vi "SECoP-Initialize.vi"(8 "error in (no error)":errorcluster, 9 "Context ID (in)":string, 10 "show status window (GUI)":bool=TRUE, 11 "DLL path (in)":path) -> (0 "error out":errorcluster, 3 "DLL path (out)":T1)   [LabVIEW 2023, in "SECoP.lvlib"]
doc: "Call <b>\"SECoP-Initialize.vi\"</b> before use of any SHALL SEC-Node related functions. This loads and initialises external SHALL libraries.\n\n<b>DLL path (in)</b> input path to directory of SHALL libraries\n<b>DLL path (out)</b>) output of cluster to be used for other VIs\n<b>show status window (GUI)</b> boolean value to <b>show</b> (true) or <b>hide</b> (false) the status window on top right corner of display"
uses:
  SECoP.lvlib
  SECoP-libraries.ctl
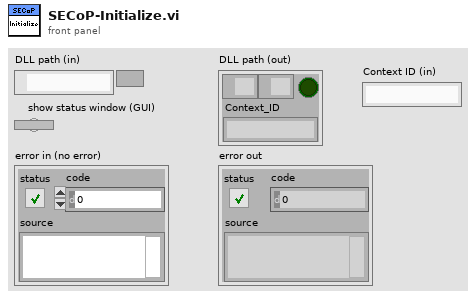
[diagram p1: front panel]
types:
  T1 = typedef "SECoP.lvlib/SECoP-libraries.ctl" = cluster{"serverDLL":path, "variantDLL":path, "cleanup_mode":bool, "Context_ID":string}
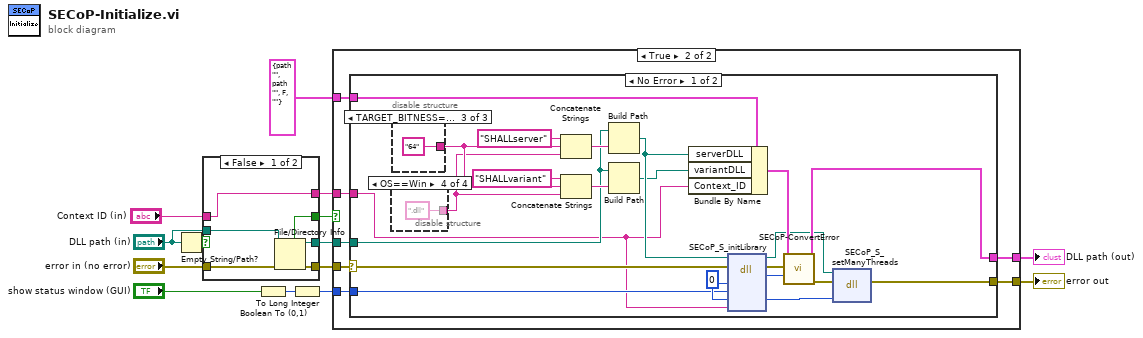
[diagram p0: block diagram]
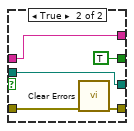
[diagram p2: hidden frame]
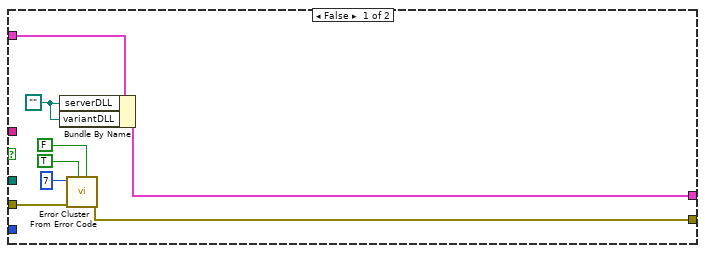
[diagram p3: hidden frame]
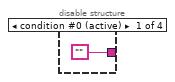
[diagram p4: hidden frame]
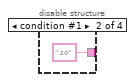
[diagram p5: hidden frame]
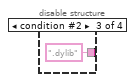
[diagram p6: hidden frame]
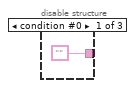
[diagram p7: hidden frame]
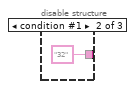
[diagram p8: hidden frame]
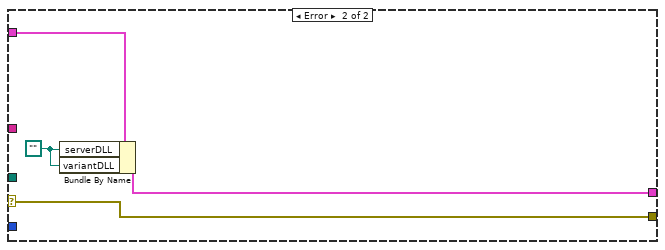
[diagram p9: hidden frame]
diagram:
  n1 = Empty String/Path?(string/path="DLL path (in)") -> (empty?=w13:bool)
  n2 = case shown="False" w13 {
    tunnel: "error in (no error)" -> [w20 w25]
    tunnel: [w19 w24] -> w8
    tunnel: "DLL path (in)" -> [w16 w22]
    tunnel: [w18 TRUE ("directory")] -> w6
    tunnel: [w17 w22] -> w5
    tunnel: "Context ID (in)" -> [w15 w21]
    tunnel: [w15 w21] -> w1
    frame False {
      n3 = File/Directory Info(path=w16, error in=w20) -> (path out=w17:path, directory=w18:bool, error out=w19:errorcluster)  [unwired: 4 out]
    }
    frame True {
      n4 = call <vilib>:"Clear Errors.vi"("error in (no error)"=w25) -> ("error out"=w24:errorcluster)  [unwired: 5 in, 1 out]
    }
  }
  n5 = Boolean To (0,1)(Boolean="show status window (GUI)") -> (0, 1=w10:i16)
  n6 = To Long Integer(number=w10) -> (32bit integer=w9:i32)
  n7 = case shown="True" w6 {
    tunnel: [w26 w40] -> w3
    tunnel: [w29 w39] -> w14
    tunnel: w9 -> [_ w38]
    tunnel: w8 -> [w33 w37]
    tunnel: w5 -> [_ w36]
    tunnel: T1 {"serverDLL"=path "", "variantDLL"=path "", "cleanup_mode"=FALSE, "Context_ID"=""} ("DLL path (out)") -> [w28 w35]
    tunnel: w1 -> [_ w34]
    frame False {
      w27 = path ""
      n8 = Bundle By Name(cluster=w28, "serverDLL"=w27, "variantDLL"=w27) -> (w26:T1)
      n9 = call <vilib>:"Error Cluster From Error Code.vi"("is warning? (False)"=FALSE, "show call chain? (False)"=TRUE, "error in (no error)"=w33, "error code (0)"=7) -> ("error out"=w29:errorcluster)  [unwired: 5 in]
    }
    frame True {
      n10 = case shown="No Error" w37 {
        selector: w37 -> [w62 w73]
        tunnel: [w47 w70] -> w40
        tunnel: [w44 w73] -> w39
        tunnel: w38 -> [w58 _]
        tunnel: w36 -> [w51 _]
        tunnel: w35 -> [w50 w71]
        tunnel: w34 -> [w41 _]
        frame No Error {
          w59 = 0 ("pApplication")
          n11 = disable-structure shown="OS==Win" {
            disable-tunnel: ["" ".so" ".dylib" ".dll"] -> w54
            frame condition #0 (active) {
            }
            frame condition #1 {
            }
            frame condition #2 {
            }
            frame condition #3 {
            }
          }
          n12 = disable-structure shown="TARGET_BITNESS==64" {
            disable-tunnel: ["" "32" "64"] -> w55
            frame condition #0 {
            }
            frame condition #1 {
            }
            frame condition #2 (active) {
            }
          }
          n13 = Concatenate Strings("SHALLserver" ("string"), w55, w54) -> (w53:string)
          n14 = Concatenate Strings("SHALLvariant" ("string"), w55, w54) -> (w52:string)
          n15 = Build Path(base path=w51, name or relative path=w53) -> (appended path=w49:path)
          n16 = Build Path(base path=w51, name or relative path=w52) -> (appended path=w42:path)
          n17 = Bundle By Name(cluster=w50, "serverDLL"=w49, "variantDLL"=w42, "Context_ID"=w41) -> (w48:T1)
          n18 = dll-call lib="Z:/Praktische Aufgaben/SECoP-LabVIEW2015/32bit/SECoP32.dll" fn="SECoP_S_initLibrary"(path in=w49, error in=w62, "pApplication"=w59, "bShowGUI"=w58, "bEnableFunctionPointers"=w59, "szContextID"=w41) -> (path out=w46:path, error out=w61:errorcluster, "return type"=w60:i32, "bEnableFunctionPointers"=w43:i32)  [unwired: 4 in]
          n19 = call "SECoP-ConvertError.vi"("return code"=w60, "error in (no error)"=w61, "DLL path (in)"=w48) -> ("error out"=w45:errorcluster, "DLL path (out)"=w47:T1)  [unwired: 7 in]
          n20 = dll-call lib="Z:/Praktische Aufgaben/SECoP-LabVIEW2015/32bit/SECoP32.dll" fn="SECoP_S_setManyThreads"(path in=w46, error in=w45, "bManyThreads"=w43) -> (error out=w44:errorcluster)  [unwired: 3 in, 1 out]
        }
        frame Error {
          w72 = path ""
          n21 = Bundle By Name(cluster=w71, "serverDLL"=w72, "variantDLL"=w72) -> (w70:T1)
        }
      }
    }
  }
  "DLL path (out)" <- w3
  "error out" <- w14
